vi "GetPixel.vi"(8 "error in (no error)":errorcluster, 9 "y":i32, 10 "x":i32, 11 "hdc":u32) -> (0 "error out":errorcluster, 3 "rgb":u32)   [LabVIEW 2019]
uses:
  gdi32.dll
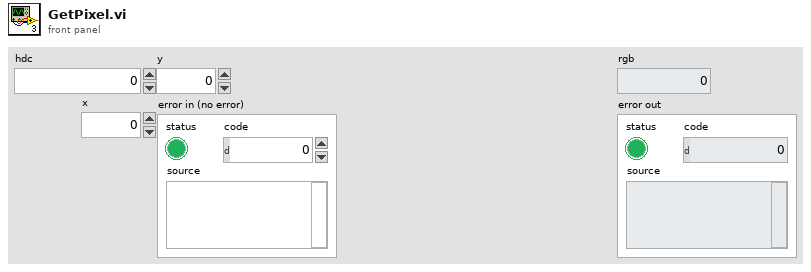
[diagram p1: front panel]
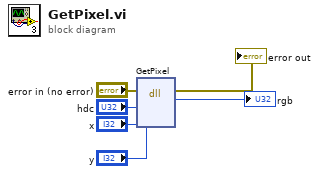
[diagram p0: block diagram]
diagram:
  n1 = dll-call lib="gdi32.dll" fn="GetPixel"(error in="error in (no error)", "hdc"="hdc", "x"="x", "y"="y") -> (error out=→"error out":errorcluster, "rgb"=→"rgb":u32)  [unwired: 5 in, 1 out]
